vi "User Event Abort.vi"(8 "error in (no error)":errorcluster, 11 "Action":T1=enum."Destroy") -> (0 "error out":errorcluster, 3 "User Event out":refnum<user-event>)   [LabVIEW 2014]
uses:
  User Event Action.ctl
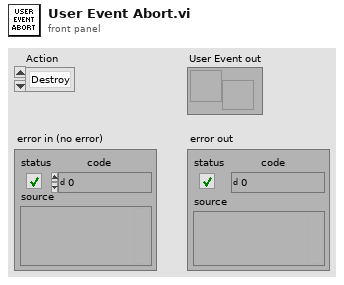
[diagram p1: front panel]
types:
  T1 = typedef "User Event Action.ctl" = enum16{"Get", "Create", "Destroy"}
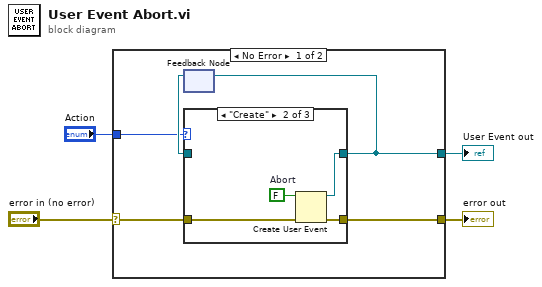
[diagram p0: block diagram]
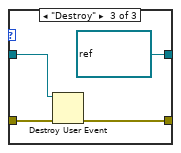
[diagram p3: hidden frame]
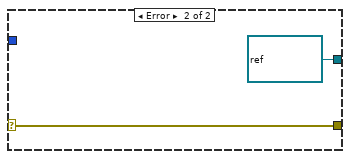
[diagram p4: hidden frame]
diagram:
  n1 = case shown="No Error" "error in (no error)" {
    selector: "error in (no error)" -> [w7 w21]
    tunnel: "Action" -> [w8 _]
    tunnel: [w6 w21] -> w3
    tunnel: [w5 refnum<user-event> refnum ("user event")] -> w4
    frame No Error {
      n2 = feedback #1() -> (w9:refnum<user-event>)  [unwired: 1 in]
      n3 = case shown="\"Create\"" w8 {
        tunnel: [w10 w15 w16] -> w6
        tunnel: [w11 w14 refnum<user-event> refnum ("user event")] -> w5
        tunnel: w9 -> [w11 _ w19]
        tunnel: w7 -> [w10 w13 w17]
        frame "Get" {
        }
        frame "Create" {
          w12 = FALSE  # Abort
          n4 = Create User Event(user event datatype=w12, error in=w13) -> (user event=w14:refnum<user-event>, error out=w15:errorcluster)
        }
        frame "Destroy" {
          n5 = Destroy User Event(user event=w19, error in=w17) -> (error out=w16:errorcluster)
        }
      }
      n6 = feedback-in #1(w5) -> ()
    }
    frame Error {
    }
  }
  "error out" <- w3
  "User Event out" <- w4
